vi "2.vi"() -> ()   [LabVIEW 2023]
panel:
  out "Waveform Chart":cluster{dbl, dbl, dbl, dbl}(graph)
  in  "Minim":dbl
  in  "Maxim":dbl
  in  "stop":bool
  in  "LN":bool
  in  "COS":bool
  in  "SIN":bool
  in  "Aleator":bool
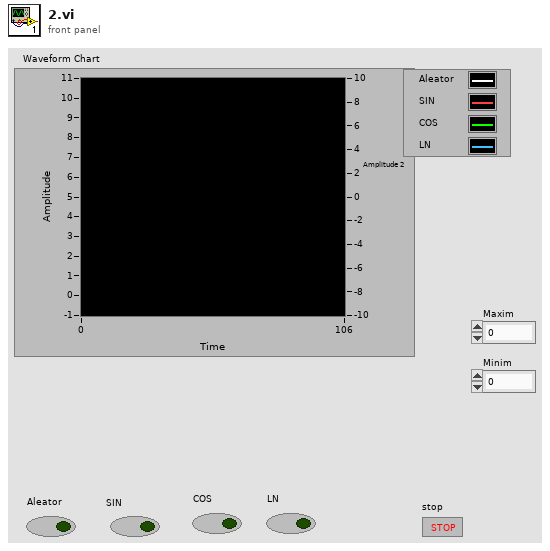
[diagram p1: front panel]
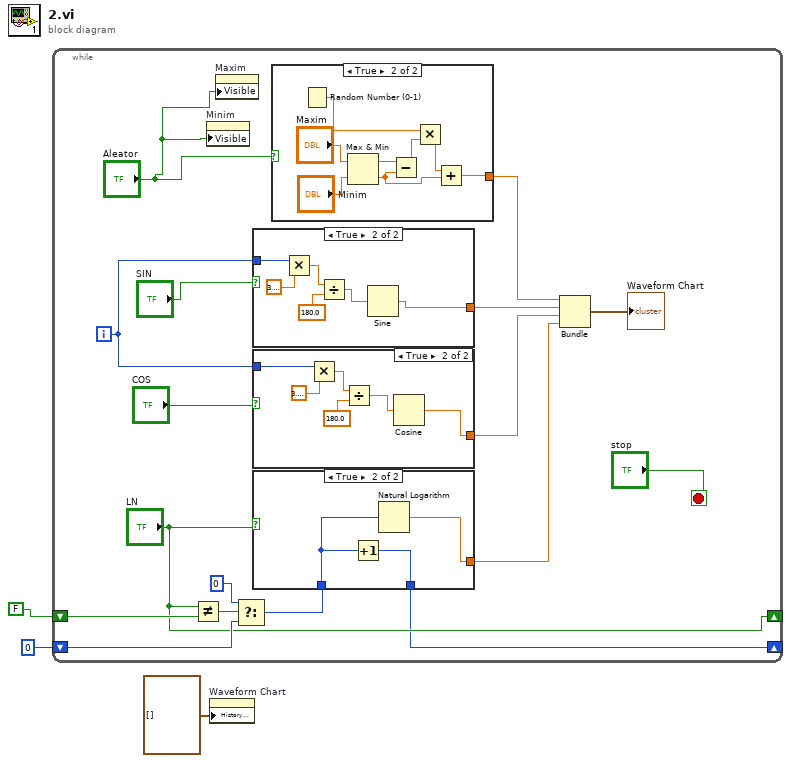
[diagram p0: block diagram]
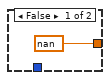
[diagram p2: hidden frame]
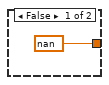
[diagram p3: hidden frame]
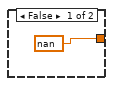
[diagram p4: hidden frame]
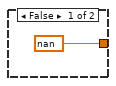
[diagram p5: hidden frame]
diagram:
  n1 = while {
    shift-right: [w7] -> _
    shift-left: 0 -> [w11]
    shift-right: ["LN"] -> _
    shift-left: FALSE -> [w9]
    i -> [w13]
    stop <- "stop" stop-if-true
    n2 = Not Equal?(x="LN", y=w9) -> (x != y?=w12:bool)
    n3 = property on="Minim" class="DigNum (strict)"("Visible"="Aleator") -> ()  [unwired: 2 in, 2 out]
    n4 = property on="Maxim" class="DigNum (strict)"("Visible"="Aleator") -> ()  [unwired: 2 in, 2 out]
    n5 = Select(t=0, s=w12, f=w11) -> (s? t:f=w6:i32)
    n6 = case shown="True" "SIN" {
      tunnel: [nan w37] -> w16
      tunnel: w13 -> [_ w34]
      frame False {
      }
      frame True {
        n7 = Multiply(x=w34, y=3.141592653589793) -> (x*y=w36:dbl)
        n8 = Divide(x=w36, y=180.0) -> (x/y=w38:dbl)
        n9 = Sine(x=w38) -> (sin(x)=w37:dbl)
      }
    }
    n10 = case shown="True" "COS" {
      tunnel: [nan w26] -> w15
      tunnel: w13 -> [_ w28]
      frame False {
      }
      frame True {
        n11 = Multiply(x=w28, y=3.141592653589793) -> (x*y=w31:dbl)
        n12 = Divide(x=w31, y=180.0) -> (x/y=w27:dbl)
        n13 = Cosine(x=w27) -> (cos(x)=w26:dbl)
      }
    }
    n14 = case shown="True" "LN" {
      tunnel: [nan w24] -> w14
      tunnel: [_ w23] -> w7
      tunnel: w6 -> [_ w22]
      frame False {
      }
      frame True {
        n15 = Increment(x=w22) -> (x+1=w23:i32)
        n16 = Natural Logarithm(1:w22) -> (0:w24:dbl)
      }
    }
    n17 = case shown="True" "Aleator" {
      tunnel: [nan w45] -> w17
      frame False {
      }
      frame True {
        n18 = Random Number (0-1)() -> (number: 0 to 1=w43:dbl)
        n19 = Max & Min(x="Maxim", y="Minim") -> (max(x,y)=w44:dbl, min(x,y)=w40:dbl)
        n20 = Subtract(x=w44, y=w40) -> (x-y=w42:dbl)
        n21 = Multiply(x=w43, y=w42) -> (x*y=w41:dbl)
        n22 = Add(x=w41, y=w40) -> (x+y=w45:dbl)
      }
    }
    n23 = Bundle "Bundle"(w17, w16, w15, w14) -> (→"Waveform Chart":cluster{dbl, dbl, dbl, dbl})  [unwired: 1 in]
  }
  n24 = property on="Waveform Chart" class="WFChart (strict)"("History Data"=cluster{dbl, dbl, dbl, dbl}[] []) -> ()  [unwired: 2 in, 2 out]
